vi "Remove Port.vi"(8 "error in":errorcluster, 11 "port ref":T1 format="%.0x") -> (0 "error out":errorcluster)   [LabVIEW 2020, in "Ballard ARINC 429 Scripting.lvlib"]
uses:
  Ballard ARINC 429 Scripting.lvlib
  <vilib>/NI VeriStand/Custom Device API/Custom Device Item Ref.ctl
  <vilib>/NI VeriStand/Custom Device API/Custom Device API.lvlib
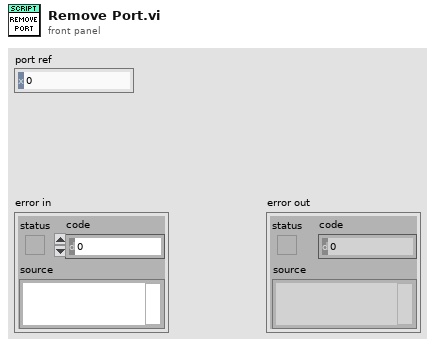
[diagram p1: front panel]
types:
  T1 = typedef "Custom Device API.lvlib/Custom Device Item Ref.ctl" = u64
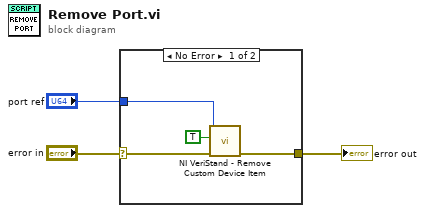
[diagram p0: block diagram]
diagram:
  n1 = case shown="No Error" "error in" {
    selector: "error in" -> [w6 w8]
    tunnel: "port ref" -> [w4 _]
    tunnel: [w7 w8] -> w2
    frame No Error {
      n2 = call <vilib>:"NI VeriStand - Remove Custom Device Item.vi"("error in (no error)"=w6, "Force Delete (F)"=TRUE, "Item Ref in"=w4) -> ("error out"=w7:errorcluster)  [unwired: 7 in, 1 out]
    }
    frame Error {
    }
  }
  "error out" <- w2
